vi "RunJavaScript.vi"(0 "reference in":refnum<class "DP_WebView.lvclass">, 1 "Java Script Function":string="document.documentElement.outerHTML", 5 "Error In":errorcluster) -> (14 "reference out":refnum<class "DP_WebView.lvclass">, 15 "Result":string, 16 "Status":i32(ring) items=["Created", "WaitingForActivation", "WaitingToRun", "Running", "WaitingForChildrenToComplete", "RanToCompletion", "Canceled", "Faulted"], 19 "Error Out":errorcluster)   [LabVIEW 2020, in "DP_WebView.lvclass"]
doc: "Get HTML comtent"
uses:
  DP_WebView.lvclass
  C:/Projects/DependencyViewer/DependencyViewer/DP_WebView_class/data/Microsoft.Web.WebView2.Core.dll
  data/Microsoft.Web.WebView2.Core.dll
  ctrls/ErrorCode.ctl
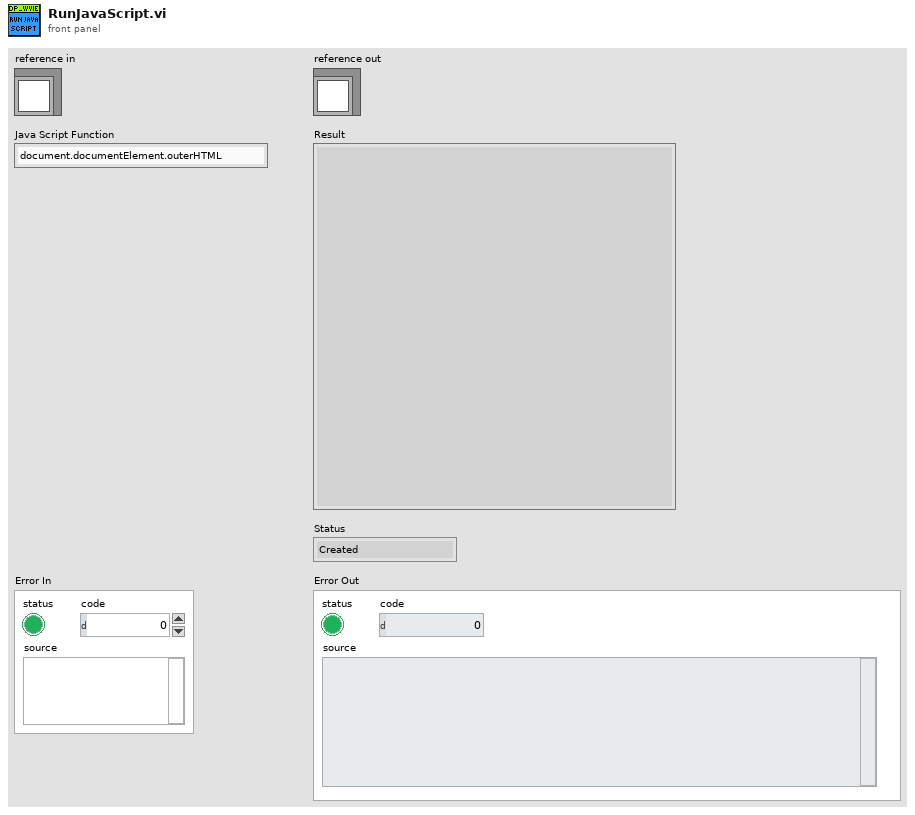
[diagram p1: front panel]
types:
  T1 = typedef "DP_WebView.lvclass/ErrorCode.ctl" = enum16{"Runtime engine is not installed or incompatible", "User Data Folder cannot be set", "Others", "JavaScript call failed", "PDF Printing Issue"}
  T2 = typedef "DP_WebView.lvclass/ObjectAttributes.ctl" = cluster{"WebView Container":refnum<k24>, "CoreWebViewRef":refnum<k24>, "Status":i32, "Status Message":string, "User Data Folder":path, "BrowserProcessId":u32}
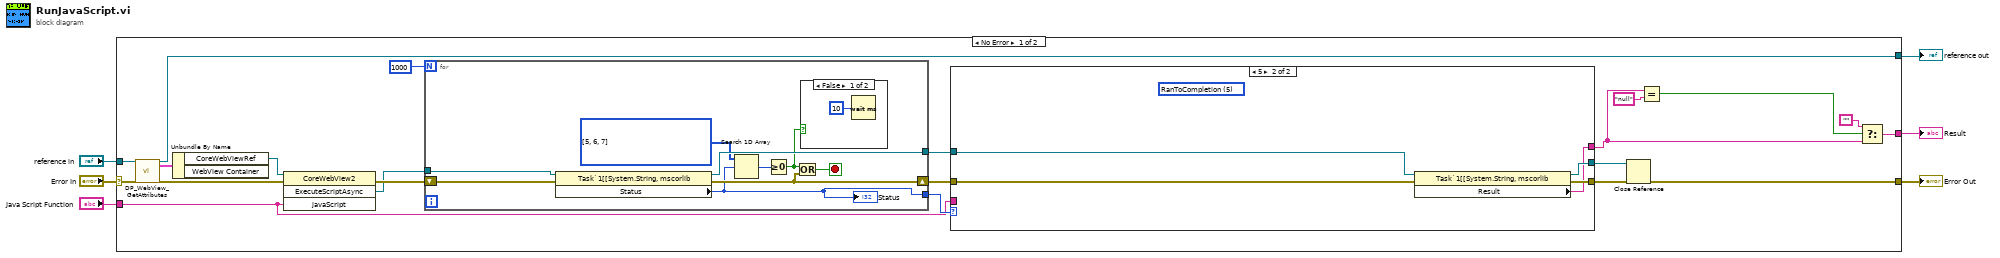
[diagram p0: block diagram]
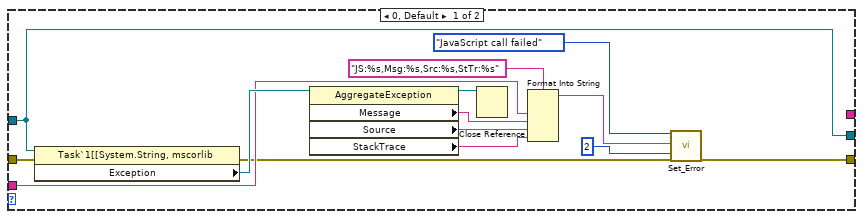
[diagram p2: hidden frame]
diagram:
  n1 = case shown="No Error" "Error In" {
    selector: "Error In" -> [w27 w58]
    tunnel: [w16 w58] -> w5
    tunnel: [w24 w57] -> w3
    tunnel: "reference in" -> [w25 w57]
    tunnel: [w12 _] -> w2
    tunnel: "Java Script Function" -> [w8 _]
    frame No Error {
      n2 = call "DP_WebView_GetAttributes.vi"("reference in"=w25, "error in (no error)"=w27) -> ("reference out"=w24:refnum<class "DP_WebView.lvclass">, "Data"=w26:T2, "error out"=w23:errorcluster)  [unwired: 14 in, 1 out]
      n3 = Unbundle By Name(w26) -> ("CoreWebViewRef"=w10:refnum<k24>)  [unwired: 1 out]
      n4 = invoke class="CoreWebView2" method="ExecuteScriptAsync"(reference=w10, error in=w23, "javaScript"=w8) -> (error out=w22:errorcluster, "ExecuteScriptAsync"=w11:refnum<k24>)  [unwired: 1 in, 2 out]
      n5 = for {
        N: 1000 -> [_]
        tunnel: w11 -> [w55]
        shift-right: [w49] -> w19
        shift-left: w22 -> [w54]
        tunnel: [w53] -> w20
        tunnel: [w47] -> w9
        stop <- w48 stop-if-true
        w52 = i32[] [5, 6, 7] items=["Created", "WaitingForActivation", "WaitingToRun", "Running", "WaitingForChildrenToComplete", "RanToCompletion", "Canceled", "Faulted"] ("Status")
        n6 = property class="Task`1[[System.String, mscorlib"(reference=w55, error in=w54) -> (reference out=w53:refnum<k24>, error out=w49:errorcluster, "Status"=w47:i32)
        "Status" <- w47
        n7 = Search 1D Array(1D array=w52, element=w47) -> (index of element=w51:i32)  [unwired: 1 in]
        n8 = Greater Or Equal To 0?(x=w51) -> (x >= 0?=w50:bool)
        n9 = Or(x=w50, y=w49) -> (x .or. y?=w48:bool)
        n10 = case shown="False" w50 {
          frame False {
            n11 = Wait (ms)(milliseconds to wait=u32 10) -> ()  [unwired: 1 out]
          }
          frame True {
          }
        }
      }
      n12 = case shown="5" w9 {
        tunnel: w20 -> [w38 w46]
        tunnel: w19 -> [w37 w45]
        tunnel: [w38 w44] -> w18
        tunnel: [w41 w43] -> w17
        tunnel: [_ w42] -> w7
        tunnel: w8 -> [w34 _]
        frame 0, Default {
          n13 = property class="Task`1[[System.String, mscorlib"(reference=w38, error in=w37) -> (error out=w29:errorcluster, "Exception"=w36:refnum<k24>)  [unwired: 1 out]
          n14 = property class="AggregateException"(reference=w36) -> (reference out=w28:refnum<k24>, "Message"=w33:string, "Source"=w32:string, "StackTrace"=w31:string)  [unwired: 1 in, 1 out]
          n15 = Close Reference(reference=w28) -> ()  [unwired: 1 in, 1 out]
          n16 = Format Into String(format string="JS:%s,Msg:%s,Src:%s,StTr:%s", w34, w33, w32, w31) -> (resulting string=w30:string)  [unwired: 2 in, 1 out]
          n17 = call "Set_Error.vi"("CustomErrors"=ErrorCode."JavaScript call failed", "Description"=w30, "Error SubVI Level(1)"=2, "error in (no error)"=w29) -> ("error out"=w41:errorcluster)  [unwired: 15 in]
        }
        frame 5 {
          (unwired) 5 items=["Created", "WaitingForActivation", "WaitingToRun", "Running", "WaitingForChildrenToComplete", "RanToCompletion", "Canceled", "Faulted"] ("Status")
          n18 = property class="Task`1[[System.String, mscorlib"(reference=w46, error in=w45) -> (reference out=w44:refnum<k24>, error out=w43:errorcluster, "Result"=w42:string)
        }
      }
      n19 = Close Reference(reference=w18, error in (no error)=w17) -> (error out=w16:errorcluster)
      n20 = Equal?(x=w7, y="null") -> (x = y?=w14:bool)
      n21 = Select(t="", s=w14, f=w7) -> (s? t:f=w12:string)
    }
    frame Error {
    }
  }
  "Error Out" <- w5
  "reference out" <- w3
  "Result" <- w2
